vi "X-Y Tracking pass reference.vi"(0 "X Parameters":T2={"Number of X Steps"=200, "Max X (V)"=2.0, "Min X (V)"=-2.0}, 1 "Y Parameters":T1={"Number of Y Steps"=200, "Max Y (V)"=2.0, "Min Y (V)"=-2.0}, 2 "X Pos":dbl=100.0, 3 "Y pos":dbl=100.0, 4 "task in":refnum<k21>) -> (5 "task out 2":refnum<k21>, 7 "X Centered Voltage":dbl, 8 "Y centered Voltage":dbl, 10 "gave up?":bool)   [LabVIEW 2011]
uses:
  <vilib>/DAQmx/write.llb/DAQmx Write (Analog 2D DBL NChan NSamp).vi
  <vilib>/DAQmx/create/channels.llb/DAQmx Create Channel (AO-Voltage-Basic).vi
  <vilib>/DAQmx/miscellaneous.llb/DAQmx Fill In Error Info.vi
  <vilib>/Analysis/NI_AALPro.lvlib
panel:
  out "Waveform Graph":dbl[](graph)
  out "Cross Section Y":dbl[](graph)
  out "Center Y":dbl
  out "Cross Section X":dbl[](graph)
  out "Center X":dbl
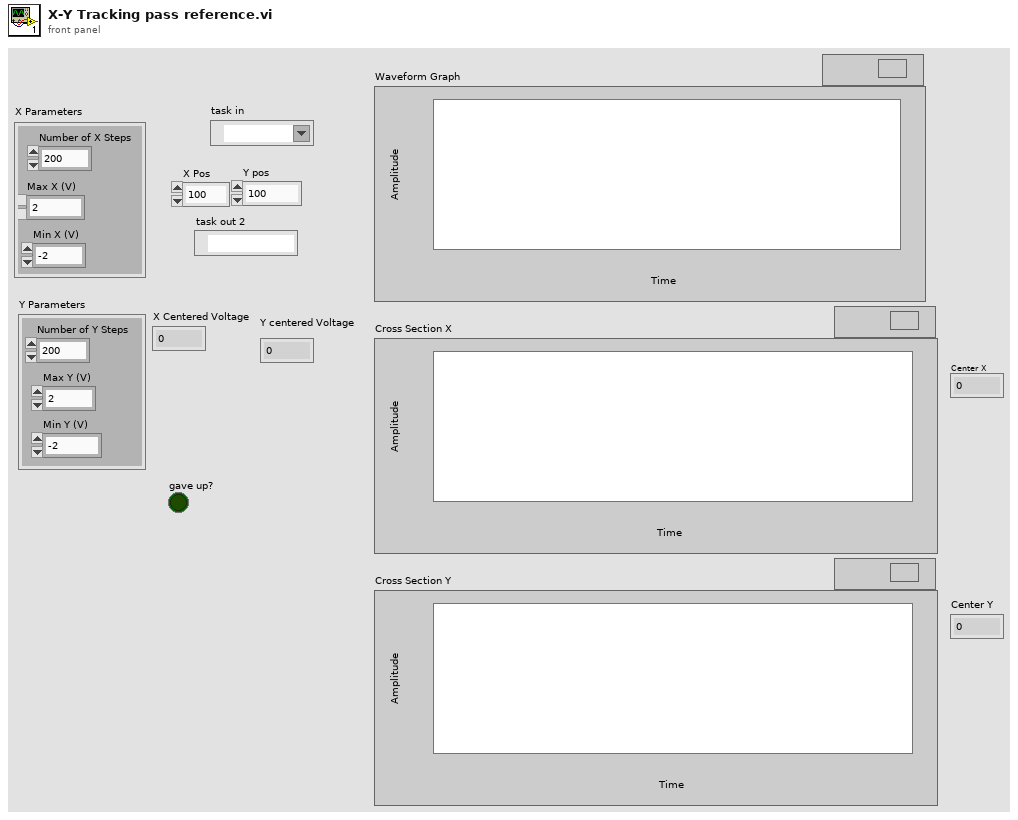
[diagram p1: front panel]
types:
  T1 = cluster{"Number of Y Steps":i32, "Max Y (V)":dbl, "Min Y (V)":dbl}
  T2 = cluster{"Number of X Steps":i32, "Max X (V)":dbl, "Min X (V)":dbl}
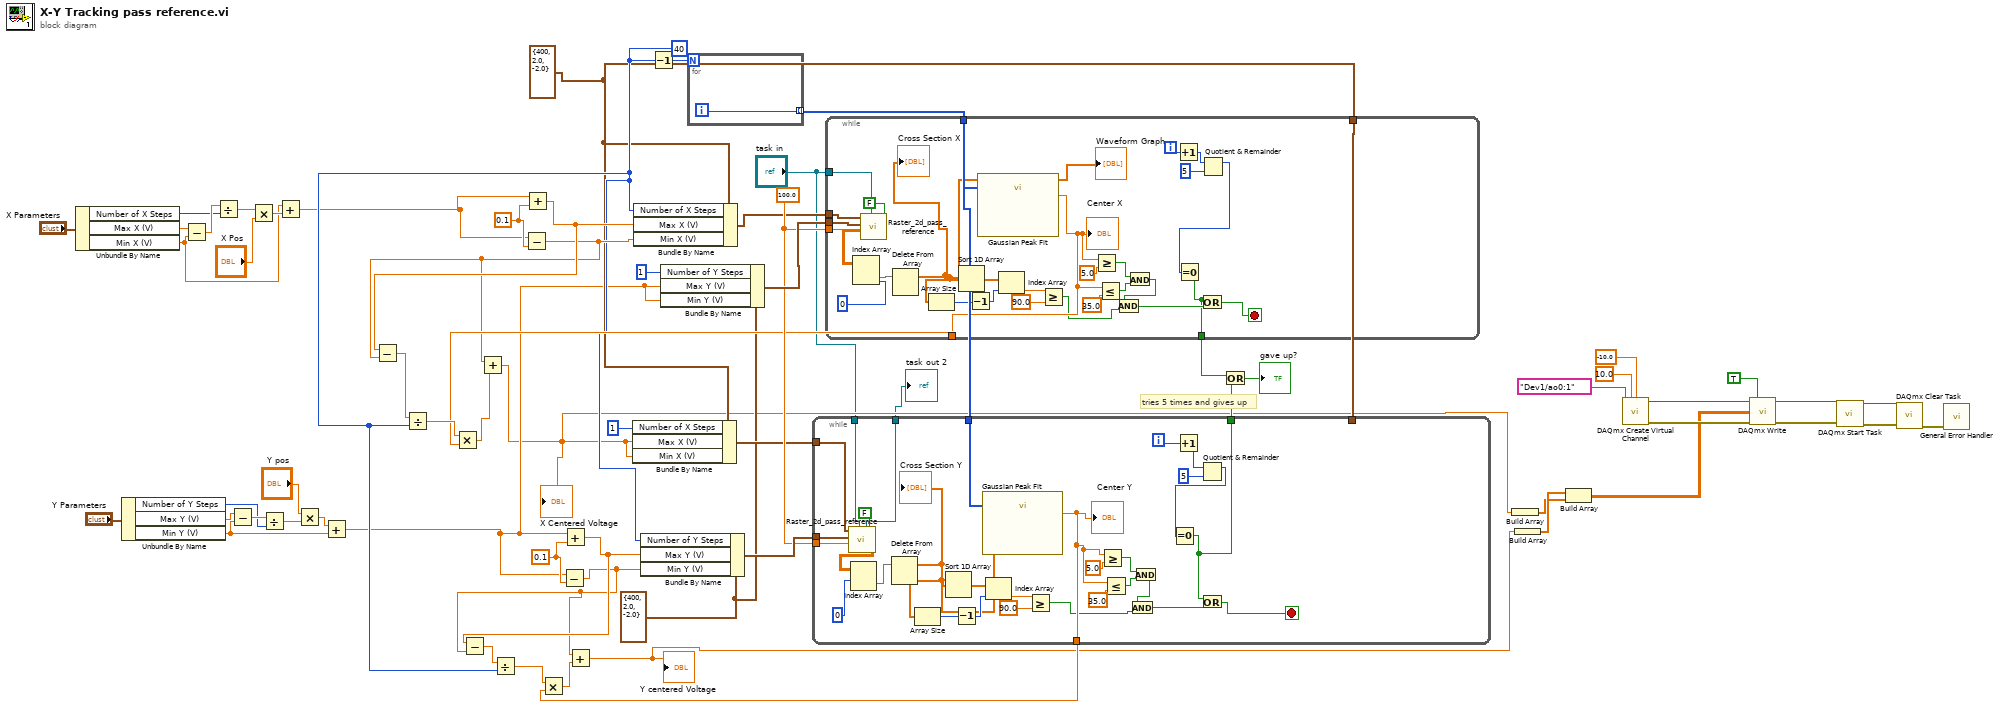
[diagram p0: block diagram]
diagram:
  w49 = 0.1 ("y")
  w50 = T1 {"Number of Y Steps"=400, "Max Y (V)"=2.0, "Min Y (V)"=-2.0} ("Y Parameters")
  w53 = 0.1 ("y")
  w41 = T2 {"Number of X Steps"=400, "Max X (V)"=2.0, "Min X (V)"=-2.0} ("X Parameters")
  w45 = 40 ("Number of X Steps")
  w60 = 100.0 ("Update Rate (Hz)")
  # "tries 5 times and gives up"
  n1 = Unbundle By Name("X Parameters") -> ("Number of X Steps"=w24:i32, "Max X (V)"=w23:dbl, "Min X (V)"=w22:dbl)
  n2 = Unbundle By Name("Y Parameters") -> ("Number of Y Steps"=w28:i32, "Max Y (V)"=w27:dbl, "Min Y (V)"=w26:dbl)
  n3 = Subtract(x=w23, y=w22) -> (x-y=w35:dbl)
  n4 = Divide(x=w35, y=w24) -> (x/y=w30:dbl)
  n5 = Subtract(x=w27, y=w26) -> (x-y=w36:dbl)
  n6 = Multiply(x=w30, y="X Pos") -> (x*y=w29:dbl)
  n7 = Divide(x=w36, y=w28) -> (x/y=w33:dbl)
  n8 = Add(x=w22, y=w29) -> (x+y=w19:dbl)
  n9 = Multiply(x="Y pos", y=w33) -> (x*y=w32:dbl)
  n10 = Add(x=w32, y=w26) -> (x+y=w20:dbl)
  n11 = Subtract(x=w19, y=w53) -> (x-y=w51:dbl)
  n12 = Add(x=w19, y=w53) -> (x+y=w52:dbl)
  n13 = Subtract(x=w52, y=w51) -> (x-y=w59:dbl)
  n14 = Divide(x=w59, y=w45) -> (x/y=w58:dbl)
  n15 = Subtract(x=w20, y=w49) -> (x-y=w42:dbl)
  n16 = Add(x=w20, y=w49) -> (x+y=w43:dbl)
  n17 = Subtract(x=w43, y=w42) -> (x-y=w48:dbl)
  n18 = Divide(x=w48, y=w45) -> (x/y=w47:dbl)
  n19 = Bundle By Name(cluster=w41, "Number of X Steps"=w45, "Max X (V)"=w52, "Min X (V)"=w51) -> (w55:T2)
  n20 = Bundle By Name(cluster=w50, "Number of Y Steps"=w45, "Max Y (V)"=w43, "Min Y (V)"=w42) -> (w62:T1)
  n21 = Decrement(x=w45) -> (x-1=w40:i32)
  n22 = Bundle By Name(cluster=w50, "Number of Y Steps"=1, "Max Y (V)"=w20, "Min Y (V)"=w20) -> (w63:T1)
  n23 = for {
    N: w40 -> [_]
    tunnel: [w66] -> w65 mode=indexing
    i -> [w66]
  }
  n24 = while {
    tunnel: w65 -> [w94]
    tunnel: w63 -> [w85]
    tunnel: w60 -> [w92]
    tunnel: [w90] -> w57
    tunnel: w55 -> [w86]
    tunnel: w41 -> [_]
    tunnel: [w68] -> w39
    tunnel: "task in" -> [w67]
    i -> [w76]
    stop <- w69 stop-if-true
    n25 = call "Raster_2d_pass_reference.vi"("Save?"=FALSE, "task in"=w67, "Update Rate (Hz)"=w92, "Y Parameters"=w85, "X Parameters"=w86) -> ("Intensity Graph"=w95:dbl[][])  [unwired: 2 in, 2 out]
    n26 = Index Array(array=w95, index (col)=0 ("index (row)")) -> (element=w73:dbl[])  [unwired: 1 in]
    n27 = Delete From Array(array=w73) -> (array with subset deleted=w72:dbl[])  [unwired: 2 in, 1 out]
    "Cross Section X" <- w72
    n28 = Array Size(array=w72) -> (size(s)=w80:i32)
    n29 = Sort 1D Array(array=w72) -> (sorted array=w84:dbl[])
    n30 = Decrement(x=w80) -> (x-1=w79:i32)
    n31 = call <vilib>:"Gaussian Peak Fit.vi"("Y"=w72, "X"=w94) -> ("Best Gaussian Fit"=→"Waveform Graph":dbl[], "center"=w90:dbl)  [unwired: 7 in, 5 out]
    "Center X" <- w90
    n32 = Index Array(array=w84, index=w79) -> (element=w83:dbl)
    n33 = Greater Or Equal?(x=w83, y=90.0) -> (x >= y?=w81:bool)
    n34 = Greater Or Equal?(x=w90, y=5.0) -> (x >= y?=w87:bool)
    n35 = Less Or Equal?(x=w90, y=35.0) -> (x <= y?=w88:bool)
    n36 = And(x=w87, y=w88) -> (x .and. y?=w75:bool)
    n37 = And(x=w75, y=w81) -> (x .and. y?=w71:bool)
    n38 = Increment(x=w76) -> (x+1=w77:i32)
    n39 = Quotient & Remainder(x=w77, y=5) -> (x-y*floor(x/y)=w70:i32)  [unwired: 1 out]
    n40 = Equal To 0?(x=w70) -> (x = 0?=w68:bool)
    n41 = Or(x=w68, y=w71) -> (x .or. y?=w69:bool)
  }
  n42 = Multiply(x=w58, y=w57) -> (x*y=w56:dbl)
  n43 = Add(x=w51, y=w56) -> (x+y=w7:dbl)
  "X Centered Voltage" <- w7
  n44 = Bundle By Name(cluster=w41, "Number of X Steps"=1 ("Number of Y Steps"), "Max X (V)"=w7, "Min X (V)"=w7) -> (w54:T2)
  n45 = while {
    tunnel: w65 -> [w126]
    tunnel: w62 -> [w117]
    tunnel: w60 -> [w125]
    tunnel: w54 -> [w118]
    tunnel: [w116] -> w44
    tunnel: w41 -> [_]
    tunnel: [w99] -> w38
    tunnel: [w98] -> w2
    tunnel: "task in" -> [w97]
    i -> [w106]
    stop <- w100 stop-if-true
    n46 = call "Raster_2d_pass_reference.vi"("Save?"=FALSE, "task in"=w97, "Update Rate (Hz)"=w125, "Y Parameters"=w117, "X Parameters"=w118) -> ("Intensity Graph"=w124:dbl[][], "task out"=w98:refnum<k21>)  [unwired: 2 in, 1 out]
    n47 = Index Array(array=w124, index (row)=0) -> (element=w103:dbl[])  [unwired: 1 in]
    n48 = Delete From Array(array=w103) -> (array with subset deleted=w102:dbl[])  [unwired: 2 in, 1 out]
    "Cross Section Y" <- w102
    n49 = Array Size(array=w102) -> (size(s)=w110:i32)
    n50 = Sort 1D Array(array=w102) -> (sorted array=w115:dbl[])
    n51 = Decrement(x=w110) -> (x-1=w109:i32)
    n52 = call <vilib>:"Gaussian Peak Fit.vi"("Y"=w102, "X"=w126) -> ("center"=w116:dbl)  [unwired: 7 in, 6 out]
    "Center Y" <- w116
    n53 = Index Array(array=w115, index=w109) -> (element=w114:dbl)
    n54 = Greater Or Equal?(x=w114, y=90.0) -> (x >= y?=w111:bool)
    n55 = Greater Or Equal?(x=w116, y=5.0) -> (x >= y?=w122:bool)
    n56 = Less Or Equal?(x=w116, y=35.0) -> (x <= y?=w121:bool)
    n57 = And(x=w122, y=w121) -> (x .and. y?=w112:bool)
    n58 = And(x=w112, y=w111) -> (x .and. y?=w101:bool)
    n59 = Increment(x=w106) -> (x+1=w105:i32)
    n60 = Quotient & Remainder(x=w105, y=5) -> (x-y*floor(x/y)=w107:i32)  [unwired: 1 out]
    n61 = Equal To 0?(x=w107) -> (x = 0?=w99:bool)
    n62 = Or(x=w99, y=w101) -> (x .or. y?=w100:bool)
  }
  "task out 2" <- w2
  n63 = Multiply(x=w47, y=w44) -> (x*y=w46:dbl)
  n64 = Add(x=w42, y=w46) -> (x+y=w6:dbl)
  "Y centered Voltage" <- w6
  n65 = Or(x=w39, y=w38) -> (x .or. y?=→"gave up?":bool)
  n66 = Build Array(w7) -> (w4:dbl[])
  n67 = Build Array(w6) -> (w5:dbl[])
  n68 = Build Array(w5, w4) -> (w3:dbl[][])
  n69 = call-poly <vilib>:"DAQmx Create Virtual Channel.vi"("maximum value"=10.0, "minimum value"=-10.0, "physical channels"=tag "Dev1/ao0:1") -> ("task out"=w15:refnum<k21>, "error out"=w14:errorcluster)  [unwired: 11 in]
  n70 = call-poly <vilib>:"DAQmx Write.vi"("task/channels in"=w15, "auto start"=TRUE, "data"=w3, "error in"=w14) -> ("task out"=w13:refnum<k21>, "error out"=w12:errorcluster)  [unwired: 9 in, 1 out]
  n71 = call <vilib>:"DAQmx Start Task.vi"("task/channels in"=w13, "error in"=w12) -> ("task out"=w11:refnum<k21>, "error out"=w10:errorcluster)  [unwired: 12 in]
  n72 = call <vilib>:"DAQmx Clear Task.vi"("task in"=w11, "error in"=w10) -> ("error out"=w9:errorcluster)  [unwired: 13 in]
  n73 = call <vilib>:"General Error Handler.vi"("error in (no error)"=w9) -> ()  [unwired: 10 in, 5 out]
